vi "Set Table Context.vi"(8 "error in (no error)":errorcluster, 9 "Context":T1, 10 "Table Names":string[](array[string]), 11 "Stack in":T1[](array[typedef])) -> (0 "error out":errorcluster, 3 "Stack out":T1[](array[typedef]))   [LabVIEW 2019, in "BlueTOMLSerializer.lvlib"]
uses:
  BlueTOMLSerializer.lvlib
  Value.ctl
  Key-Value Pair.ctl
  Table Context.ctl
  Table Array Context.ctl
  Context.ctl
  Value Type.ctl
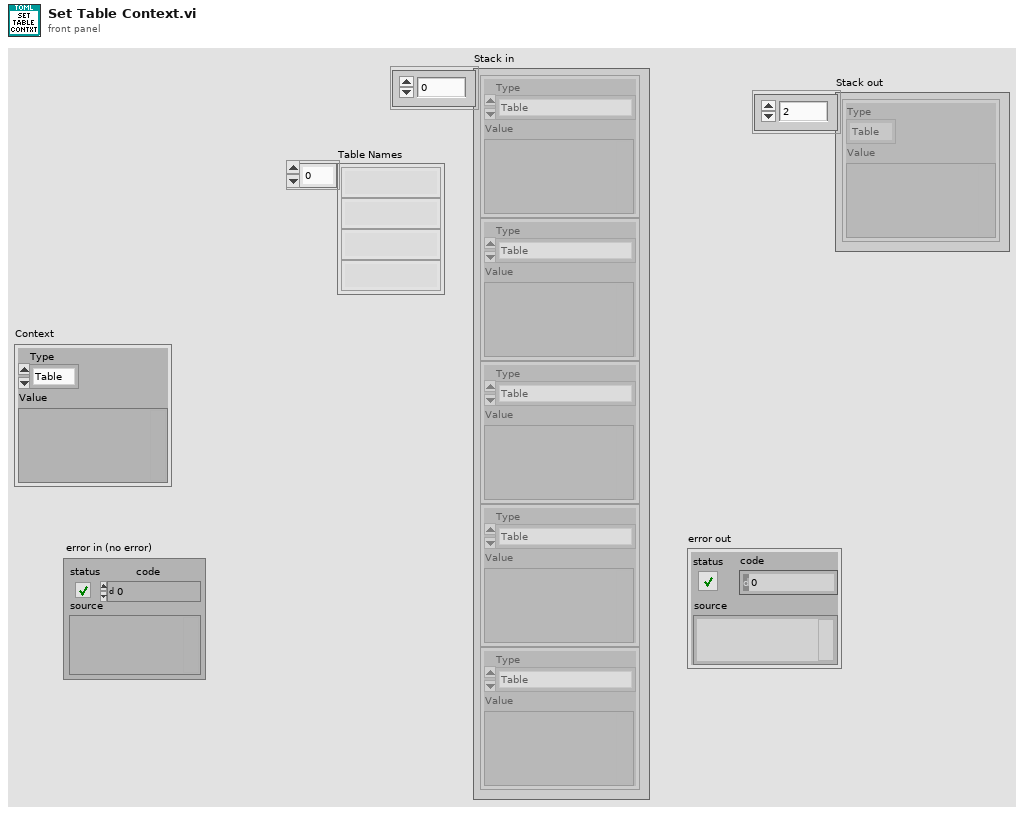
[diagram p1: front panel]
types:
  T1 = typedef "BlueTOMLSerializer.lvlib/Context.ctl" = cluster{"Type":enum16{"Table", "Array", "Inline Table", "Table Array"}, "Value":variant}
  T2 = enum16{"Table", "Array", "Inline Table", "Table Array"}
  T3 = typedef "BlueTOMLSerializer.lvlib/Value.ctl" = cluster{"Type":T4, "Value":variant}
  T4 = typedef "BlueTOMLSerializer.lvlib/Value Type.ctl" = enum16{"Table", "Array", "String", "Integer", "Float", "Boolean", "Offset Date-Time", "Local Date-Time", "Local Date", "Local Time"}
  T5 = typedef "BlueTOMLSerializer.lvlib/Table Context.ctl" = cluster{"Table":T6[], "Key":string, "Defined Keys":string[]}
  T6 = typedef "BlueTOMLSerializer.lvlib/Key-Value Pair.ctl" = cluster{"Key":string, "Value":T3}
  T7 = typedef "BlueTOMLSerializer.lvlib/Table Array Context.ctl" = cluster{"Table Array":cluster{"Table":T6[]}[], "Index":i32, "Key":string}
  T8 = typedef "TOML.lvlib/Context.ctl" = cluster{"Type":enum16{"Table", "Array", "Inline Table", "Table Array"}, "Value":variant}
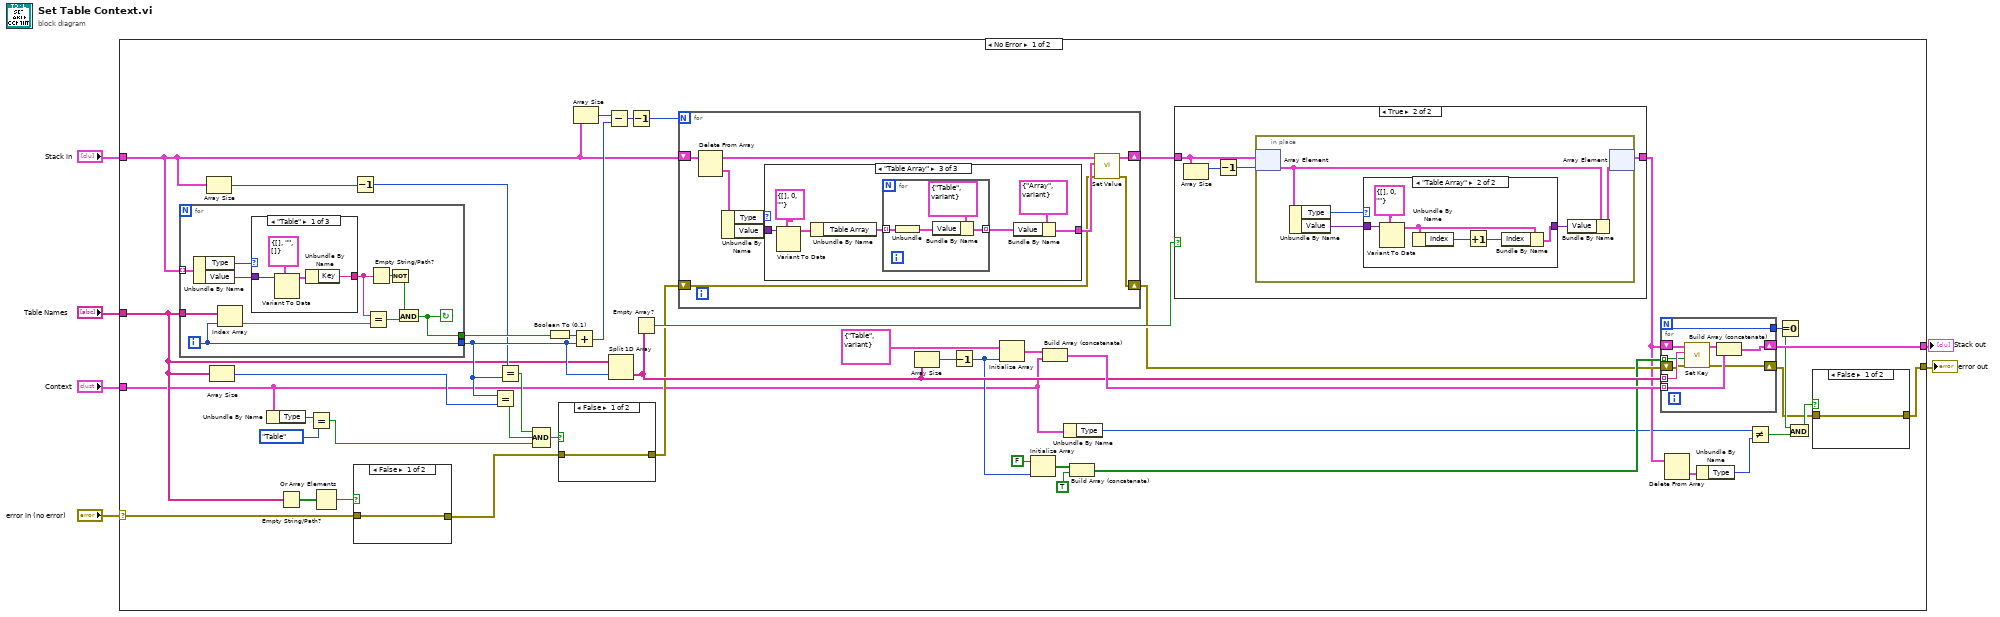
[diagram p0: block diagram]
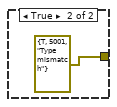
[diagram p2: hidden frame]
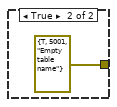
[diagram p3: hidden frame]
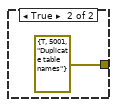
[diagram p4: hidden frame]
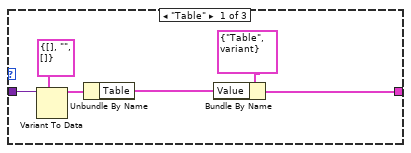
[diagram p5: hidden frame]
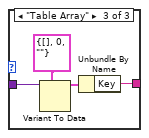
[diagram p10: hidden frame]
diagram:
  n1 = case shown="No Error" "error in (no error)" {
    selector: "error in (no error)" -> [w19 w132]
    tunnel: [w49 w133] -> w6
    tunnel: "Context" -> [w17 _]
    tunnel: [w9 w132] -> w4
    tunnel: "Table Names" -> [w22 _]
    tunnel: "Stack in" -> [w34 w133]
    frame No Error {
      n2 = for {
        tunnel: w34 -> [w122] mode=indexing
        tunnel: w22 -> [w123]
        tunnel: [w115] -> w31
        tunnel: [w114] -> w54
        i -> [w115]
        stop <- w114 continue-if-true
        n3 = Unbundle By Name(w122) -> ("Type"=w121:T2, "Value"=w120:variant)
        n4 = Index Array(array=w123, index=w115) -> (element=w119:string)
        n5 = case shown="\"Table\"" w121 {
          tunnel: w120 -> [w127 _ w131]
          tunnel: [w124 _ w128] -> w118
          frame "Table" {
            n6 = Variant To Data(type=T5 {"Table"=[], "Key"="", "Defined Keys"=[]} ("Table Context"), Variant=w127) -> (data=w125:T5)  [unwired: 1 in, 1 out]
            n7 = Unbundle By Name(w125) -> ("Key"=w124:string)
          }
          frame Default {
          }
          frame "Table Array" {
            n8 = Variant To Data(type=T7 {"Table Array"=[], "Index"=0, "Key"=""} ("Table Array Context"), Variant=w131) -> (data=w129:T7)  [unwired: 1 in, 1 out]
            n9 = Unbundle By Name(w129) -> ("Key"=w128:string)
          }
        }
        n10 = Equal?(x=w118, y=w119) -> (x = y?=w117:bool)
        n11 = Empty String/Path?(string/path=w118) -> (empty?=w116:bool)
        n12 = Not(x=w116) -> (.not. x?=w113:bool)
        n13 = And(x=w113, y=w117) -> (x .and. y?=w114:bool)
      }
      n14 = Array Size(array=w34) -> (size(s)=w32:i32)
      n15 = Array Size(array=w22) -> (size(s)=w33:i32)
      n16 = Unbundle By Name(w17) -> ("Type"=w25:T2)
      n17 = Empty String/Path?(string/path=w22) -> (empty?=w21:bool[])
      n18 = Equal?(x=w25, y=T2."Table") -> (x = y?=w23:bool)
      n19 = Or Array Elements(Boolean array=w21) -> (logical OR=w7:bool)
      n20 = Decrement(x=w32) -> (x-1=w26:i32)
      n21 = case shown="False" w7 {
        tunnel: [w57 errorcluster {"status"=TRUE, "code"=5001, "source"="Empty table name"} ("error constant")] -> w20
        tunnel: w19 -> [w57 _]
        frame False {
        }
        frame True {
        }
      }
      n22 = Equal?(x=w31, y=w33) -> (x = y?=w29:bool)
      n23 = Equal?(x=w26, y=w31) -> (x = y?=w28:bool)
      n24 = Compound Arithmetic op=AND(w28, w29, w23) -> (w30:bool)
      n25 = Boolean To (0,1)(Boolean=w54) -> (0, 1=w53:i16)
      n26 = case shown="False" w30 {
        tunnel: w20 -> [w59 _]
        tunnel: [w59 errorcluster {"status"=TRUE, "code"=5001, "source"="Duplicate table names"} ("error constant")] -> w27
        frame False {
        }
        frame True {
        }
      }
      n27 = Add(x=w53, y=w31) -> (x+y=w50:i32)
      n28 = Array Size(array=w34) -> (size(s)=w52:i32)
      n29 = Subtract(x=w52, y=w50) -> (x-y=w51:i32)
      n30 = Split 1D Array(array=w22, index=w31) -> (second subarray=w43:string[])  [unwired: 1 out]
      n31 = Decrement(x=w51) -> (x-1=w48:i32)
      n32 = Empty Array?(array=w43) -> (empty?=w41:bool)
      n33 = for {
        N: w48 -> [_]
        shift-right: [w64] -> w42
        shift-left: w34 -> [w69]
        shift-right: [w61] -> w35
        shift-left: w27 -> [w62]
        n34 = Delete From Array(array=w69) -> (deleted portion=w66:T1, array with subset deleted=w65:T1[])  [unwired: 2 in]
        n35 = Unbundle By Name(w66) -> ("Type"=w67:T2, "Value"=w68:variant)
        n36 = case shown="\"Table Array\"" w67 {
          tunnel: w68 -> [w75 _ w82]
          tunnel: [w70 _ w76] -> w63
          frame "Table" {
            n37 = Variant To Data(type=T5 {"Table"=[], "Key"="", "Defined Keys"=[]} ("Table Context"), Variant=w75) -> (data=w73:T5)  [unwired: 1 in, 1 out]
            n38 = Unbundle By Name(w73) -> ("Table"=w71:T6[])
            n39 = Bundle By Name(cluster=T3 {"Type"=enum."Table", "Value"=variant} ("Value"), "Value"=w71) -> (w70:T3)
          }
          frame Default {
          }
          frame "Table Array" {
            n40 = Variant To Data(type=T7 {"Table Array"=[], "Index"=0, "Key"=""} ("Table Array Context"), Variant=w82) -> (data=w80:T7)  [unwired: 1 in, 1 out]
            n41 = Unbundle By Name(w80) -> ("Table Array"=w79:cluster{"Table":T6[]}[])
            n42 = for {
              tunnel: w79 -> [w86] mode=indexing
              tunnel: [w83] -> w77 mode=indexing
              n43 = Unbundle(w86) -> ("Table"=w84:T6[])
              n44 = Bundle By Name(cluster=T3 {"Type"=enum."Table", "Value"=variant} ("Value"), "Value"=w84) -> (w83:T3)
            }
            n45 = Bundle By Name(cluster=T3 {"Type"=enum."Array", "Value"=variant} ("Value"), "Value"=w77) -> (w76:T3)
          }
        }
        n46 = call "Set Value.vi"("error in (no error)"=w62, "Value"=w63, "Context in"=w65) -> ("error out"=w61:errorcluster, "Context out"=w64:T1[])  [unwired: 5 in, 2 out]
      }
      n47 = Array Size(array=w43) -> (size(s)=w47:i32)
      n48 = Decrement(x=w47) -> (x-1=w40:i32)
      n49 = Initialize Array(T1 {"Type"=enum."Table", "Value"=variant} ("Context"), w40) -> (w45:T1[])
      n50 = Initialize Array(FALSE, w40) -> (w38:bool[])
      n51 = Build Array (concatenate)(w45, w17) -> (w44:T1[])
      n52 = Unbundle By Name(w17) -> ("Type"=w13:T2)
      n53 = Build Array (concatenate)(w38, TRUE) -> (w36:bool[])
      n54 = case shown="True" w41 {
        tunnel: w42 -> [w87 w91]
        tunnel: [w87 w90] -> w16
        frame False {
        }
        frame True {
          n55 = Array Size(array=w91) -> (size(s)=w89:i32)
          n56 = Decrement(x=w89) -> (x-1=w88:i32)
          n57 = in-place {
            n58 = in-place-array #1(w91, w88) -> (w94:T1)
            n59 = Unbundle By Name(w94) -> ("Type"=w96:T2, "Value"=w95:variant)
            n60 = case shown="\"Table Array\"" w96 {
              tunnel: w95 -> [w97 w103]
              tunnel: [w97 w98] -> w93
              frame Default {
              }
              frame "Table Array" {
                n61 = Variant To Data(type=T7 {"Table Array"=[], "Index"=0, "Key"=""} ("Table Array Context"), Variant=w103) -> (data=w101:T7)  [unwired: 1 in, 1 out]
                n62 = Unbundle By Name(w101) -> ("Index"=w99:i32)
                n63 = Increment(x=w99) -> (x+1=w100:i32)
                n64 = Bundle By Name(cluster=w101, "Index"=w100) -> (w98:T7)
              }
            }
            n65 = Bundle By Name(cluster=w94, "Value"=w93) -> (w92:T1)
            n66 = in-place-array #1(w92) -> (w90:T1[])  [unwired: 1 out]
          }
        }
      }
      n67 = for {
        N -> [w104]
        shift-right: [w110] -> w49
        shift-left: w16 -> [w112]
        tunnel: w43 -> [w111] mode=indexing
        tunnel: w44 -> [w109] mode=indexing
        tunnel: w36 -> [w107] mode=indexing
        shift-right: [w105] -> w8
        shift-left: w35 -> [w106]
        tunnel: [w104] -> w18
        n68 = call "Set Key.vi"("error in (no error)"=w106, "Define"=w107, "Key"=w111, "Stack in"=w112) -> ("error out"=w105:errorcluster, "Stack out"=w108:T8[])  [unwired: 6 in]
        n69 = Build Array (concatenate)(w108, w109) -> (w110:T1[])
      }
      n70 = Delete From Array(array=w16) -> (deleted portion=w15:T1)  [unwired: 2 in, 1 out]
      n71 = Unbundle By Name(w15) -> ("Type"=w14:T2)
      n72 = Not Equal?(x=w13, y=w14) -> (x != y?=w12:bool)
      n73 = Equal To 0?(x=w18) -> (x = 0?=w11:bool)
      n74 = And(x=w11, y=w12) -> (x .and. y?=w10:bool)
      n75 = case shown="False" w10 {
        tunnel: [w55 errorcluster {"status"=TRUE, "code"=5001, "source"="Type mismatch"} ("error constant")] -> w9
        tunnel: w8 -> [w55 _]
        frame False {
        }
        frame True {
        }
      }
    }
    frame Error {
    }
  }
  "Stack out" <- w6
  "error out" <- w4
